vi "NewRequest.vi"(6 "timeout in ms (-1)":i32=-1, 8 "error in (no error)":errorcluster, 9 "String":string, 11 "module in":refnum<class "Testing.lvclass">) -> (0 "error out":errorcluster, 1 "Numeric":dbl, 3 "module out":refnum<class "Testing.lvclass">, 4 "timed out?":bool)   [LabVIEW 2024, in "Testing.lvclass"]
uses:
  Testing.lvclass
  Testing.lvclass/Testing.ctl
  JQMHCore/Module/RQMHModule.lvclass
  JQMHCore/Module/Reply.ctl
  NewRequest Args.ctl
  NewRequest ReplyArgs.ctl
  C:/DevOps/CORTEX/JQMH/JQMHCore/Module/RQMHModule.lvclass
  C:/DevOps/CORTEX/JQMH/ModuleTemplates/Testing/Testing.lvclass
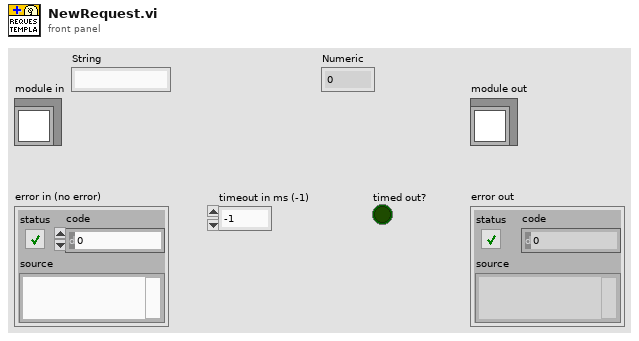
[diagram p1: front panel]
types:
  T1 = typedef "Testing.lvclass/NewRequest Args.ctl" = cluster{"String":string}
  T2 = typedef "RQMHModule.lvclass/Reply.ctl" = cluster{"Expects Reply":bool, "Reply":refnum<notifier>}
  T3 = typedef "Testing.lvclass/NewRequest ReplyArgs.ctl" = cluster{"Numeric":dbl}
  T4 = cluster{"RQMH_REPLYARGS":T3, "error in (no error)":errorcluster}
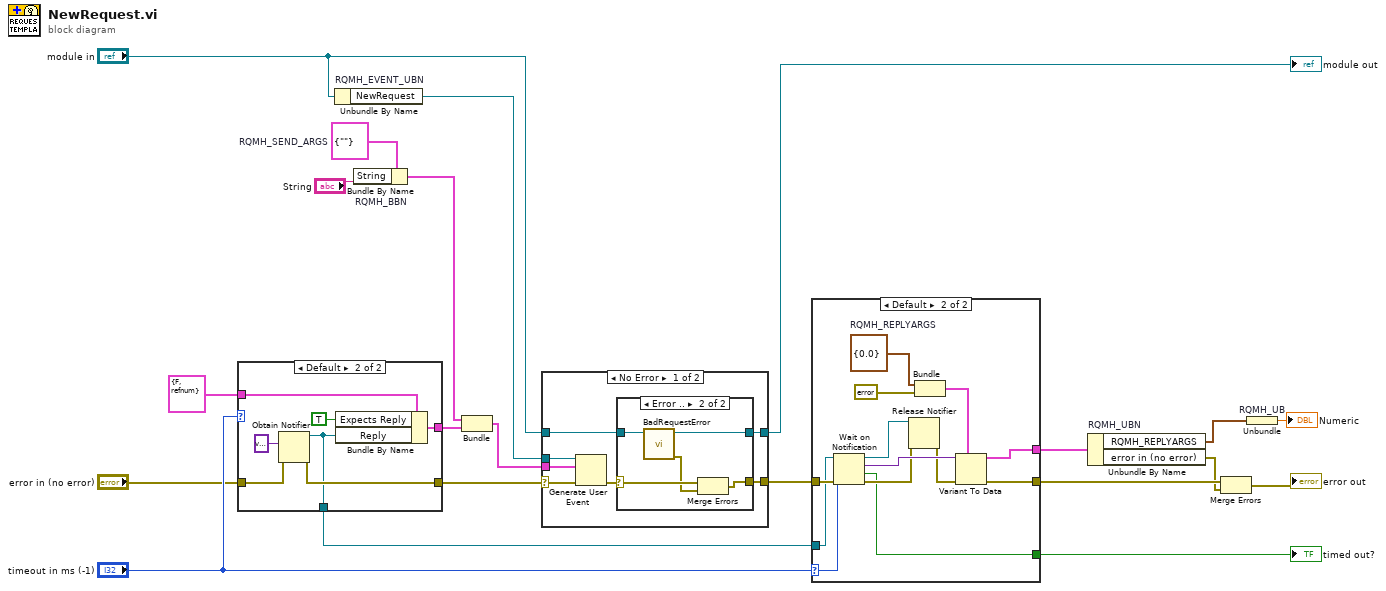
[diagram p0: block diagram]
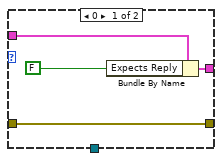
[diagram p4: hidden frame]
diagram:
  w11 = T1 {"String"=""}  # RQMH_SEND_ARGS
  n1 = case shown="Default" "timeout in ms (-1)" {
    tunnel: [w24 w31] -> w21
    tunnel: "error in (no error)" -> [w22 w30]
    tunnel: [w22 w29] -> w19
    tunnel: [_ w28] -> w17
    tunnel: T2 {"Expects Reply"=FALSE, "Reply"=refnum} ("Reply") -> [w25 w27]
    frame 0 {
      n2 = Bundle By Name(cluster=w25, "Expects Reply"=FALSE) -> (w24:T2)
    }
    frame Default {
      n3 = Obtain Notifier(notification data type=variant, error in (no error)=w30) -> (notifier out=w28:refnum<notifier>, error out=w29:errorcluster)  [unwired: 2 in, 1 out]
      n4 = Bundle By Name(cluster=w27, "Expects Reply"=TRUE, "Reply"=w28) -> (w31:T2)
    }
  }
  n5 = Unbundle By Name "RQMH_EVENT_UBN"("module in") -> ("NewRequest"=w9:refnum<user-event>)
  n6 = Bundle By Name "RQMH_BBN"(cluster=w11, "String"="String") -> (w8:T1)
  n7 = Bundle("RQMH_SEND_ARGS"=w8, "Reply"=w21) -> (w20:cluster{"RQMH_SEND_ARGS":T1, "Reply":T2})  [unwired: 1 in]
  n8 = case shown="No Error" w19 {
    selector: w19 -> [w36 w47]
    tunnel: w20 -> [w39 _]
    tunnel: w9 -> [w38 _]
    tunnel: [w35 w47] -> w18
    tunnel: "module in" -> [w34 w48]
    tunnel: [w33 w48] -> w12
    frame No Error {
      n9 = Generate User Event(user event=w38, event data cluster=w39, error in=w36) -> (error out=w37:errorcluster)  [unwired: 1 in, 1 out]
      n10 = case shown="Error .." w37 {
        selector: w37 -> [w40 w46]
        tunnel: [w40 w45] -> w35
        tunnel: w34 -> [w41 w44]
        tunnel: [w41 w43] -> w33
        frame No Error {
        }
        frame Error {
          n11 = call "BadRequestError.vi"("JQMHModule in"=w44) -> ("error out"=w42:errorcluster, "JQMHModule out"=w43:refnum<class "Testing.lvclass">)  [unwired: 9 in]
          n12 = Merge Errors(w46, w42) -> (w45:errorcluster)
        }
      }
    }
    frame Error {
    }
  }
  "module out" <- w12
  n13 = case shown="Default" "timeout in ms (-1)" {
    selector: "timeout in ms (-1)" -> [_ w53]
    tunnel: w18 -> [w49 w62]
    tunnel: w17 -> [_ w61]
    tunnel: [_ w54] -> w16
    tunnel: [w49 w51] -> w7
    tunnel: [_ w50] -> w6
    frame 0 {
    }
    frame Default {
      w52 = T3 {"Numeric"=0.0}  # RQMH_REPLYARGS
      n14 = Wait on Notification(notifier=w61, timeout in ms (-1)=w53, error in (no error)=w62) -> (notifier out=w57:refnum<notifier>, notification=w58:variant, timed out?=w54:bool, error out=w56:errorcluster)  [unwired: 1 in]
      n15 = Release Notifier(notifier=w57, error in (no error)=w56) -> (error out=w55:errorcluster)  [unwired: 1 in, 2 out]
      n16 = Bundle("RQMH_REPLYARGS"=w52, "error in (no error)"=errorcluster {"status"=FALSE, "code"=0, "source"=""}) -> (w60:T4)  [unwired: 1 in]
      n17 = Variant To Data(error in=w55, type=w60, Variant=w58) -> (data=w50:T4, error out=w51:errorcluster)
    }
  }
  "timed out?" <- w16
  n18 = Unbundle By Name "RQMH_UBN"(w6) -> ("RQMH_REPLYARGS"=w3:T3, "error in (no error)"=w4:errorcluster)
  n19 = Merge Errors(w7, w4) -> (→"error out":errorcluster)
  n20 = Unbundle "RQMH_UB"(w3) -> ("Numeric"=→"Numeric":dbl)
